vi "Receive Value Change Event.vi"(8 "error in (no error)":errorcluster, 10 "ValueChangeMsg":refnum<class "ValueChangeMsg.lvclass">, 11 "TopButton In":refnum<class "TopButton.lvclass">) -> (0 "error out":errorcluster, 3 "TopButton Out":refnum<class "TopButton.lvclass">)   [LabVIEW 2017, in "TopButton.lvlib" / "TopButton.lvclass"]
doc: "<License>\nCopyright © 2017 Composed Systems, LLC | All rights reserved\nwww.composed.io\n\nAuthor: Ethan Stern <ethan.stern@composed.io>\n\nThis software is provided \"AS IS\" WITHOUT WARRANTIES, either express or implied, AND IS FOR EDUCATIONAL PURPOSES ONLY.\n</License>"
uses:
  <vilib>/gpm_packages/TestSystem/Views/TopButton/TopButton/TopButton.lvclass
  <vilib>/gpm_packages/@cs/mva-viewable/Source/ActorEvents/IEventAggregator Messages/ValueChangeMsg/ValueChangeMsg.lvclass
  <vilib>/gpm_packages/@cs/mva-viewable/Source/ActorEvents/IEventAggregator Messages/ValueChangeMsg/ValueChangeMsg.lvclass/ValueChangeMsg.ctl
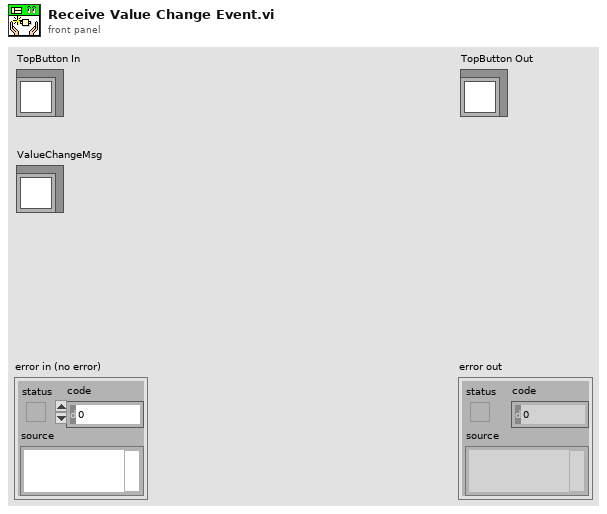
[diagram p1: front panel]
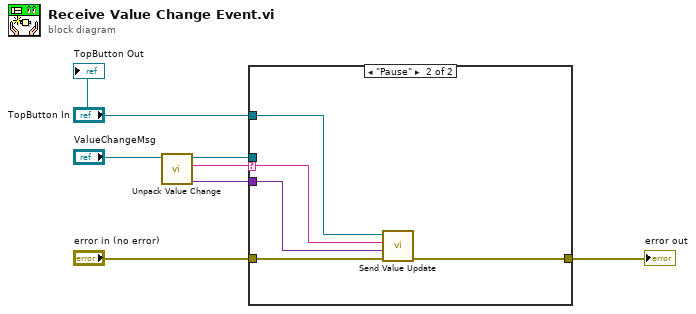
[diagram p0: block diagram]
diagram:
  n1 = call <vilib>:"Unpack Value Change.vi"("ValueChangeMsg"="ValueChangeMsg") -> ("New Value"=w4:variant, "Control Label"=w6:string, "Ctl Refnum"=w5:refnum<vi>)  [unwired: 6 in, 2 out]
  n2 = case shown="\"Pause\"" w6 {
    selector: w6 -> [_ w12]
    tunnel: "TopButton In" -> [_ w13]
    tunnel: w5 -> [_ _]
    tunnel: w4 -> [_ w11]
    tunnel: "error in (no error)" -> [w8 w10]
    tunnel: [w8 w9] -> w2
    frame "False", Default {
    }
    frame "Pause" {
      n3 = call-dynamic "Send Value Update.vi"("error in (no error)"=w10, "Value"=w11, "Datum Name"=w12, "IViewable in"=w13) -> ("error out"=w9:errorcluster)  [unwired: 7 in]
    }
  }
  "error out" <- w2
  "TopButton Out" <- "TopButton In"
